vi "create_folders_and_log.vi"(9 "Date array":string[](array[string]), 10 "Experiment title":string, 11 "Username":string) -> (2 "Data Output Folder":path, 3 "File path for master log":path)   [LabVIEW 2016]
uses:
  <vilib>/Utility/file.llb/Write Delimited Spreadsheet (string).vi
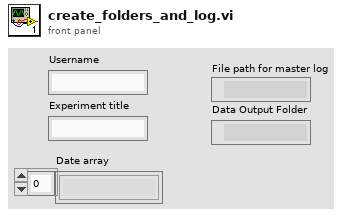
[diagram p1: front panel]
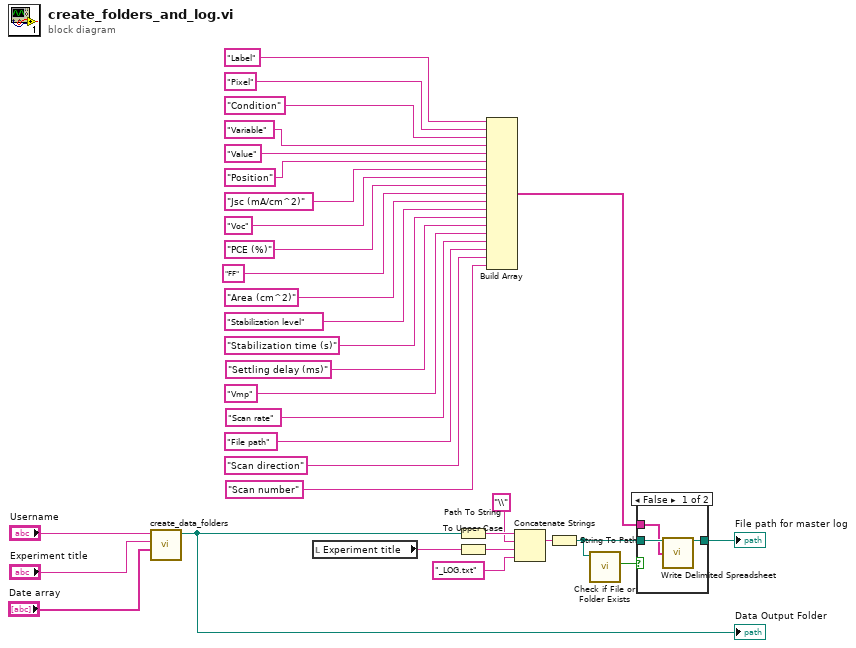
[diagram p0: block diagram]
diagram:
  n1 = call "create_data_folders.vi"("Date array"="Date array", "Experiment Indicator"="Experiment title", "username"="Username") -> ("Data Output Folder"=w3:path)  [unwired: 8 in]
  "Data Output Folder" <- w3
  n2 = local read "Experiment title"() -> (w26:string)
  n3 = Path To String(path=w3) -> (string=w33:string)
  n4 = To Upper Case(1:w26) -> (0:w27:string)
  n5 = Build Array("Label", "Pixel", "Condition", "Variable", "Value", "Position", "Jsc (mA/cm^2)", "Voc", "PCE (%)", "FF", "Area (cm^2)", "Stabilization level", "Stabilization time (s)", "Settling delay (ms)", "Vmp", "Scan rate", "File path", "Scan direction", "Scan number") -> (w9:string[])
  n6 = Concatenate Strings(w33, "\\", w27, "_LOG.txt") -> (w31:string)
  n7 = String To Path(string=w31) -> (path=w1:path)
  n8 = call <vilib>:"Check if File or Folder Exists.vi"("path"=w1) -> ("file or folder exists?"=w10:bool)  [unwired: 8 in, 2 out]
  n9 = case shown="False" w10 {
    tunnel: w1 -> [w36 w37]
    tunnel: [w35 w37] -> w2
    tunnel: w9 -> [w34 _]
    frame False {
      n10 = call-poly <vilib>:"Write Delimited Spreadsheet.vi"("file path (dialog if empty)"=w36, "1D data"=w34) -> ("new file path (Not A Path if cancelled)"=w35:path)  [unwired: 12 in, 1 out]
    }
    frame True {
    }
  }
  "File path for master log" <- w2
